vi "MTMount_getNextSample_OSS6.vi"(8 "error in (no error)":errorcluster, 11 "OSS6_Ctl":T1) -> (0 "error out":errorcluster, 2 "function return":i32, 3 "OSS6_Ctl out":T1)   [LabVIEW 2018, in "SALLV_MTMount.lvlib"]
doc: "int MTMount_shm_getNextSample_OSS6LV(MTMount_OSS6LV *OSS6_Ctl );"
uses:
  SALLV_MTMount.lvlib
  DataTypes/OSS6.ctl
  SALLV_MTMount.so
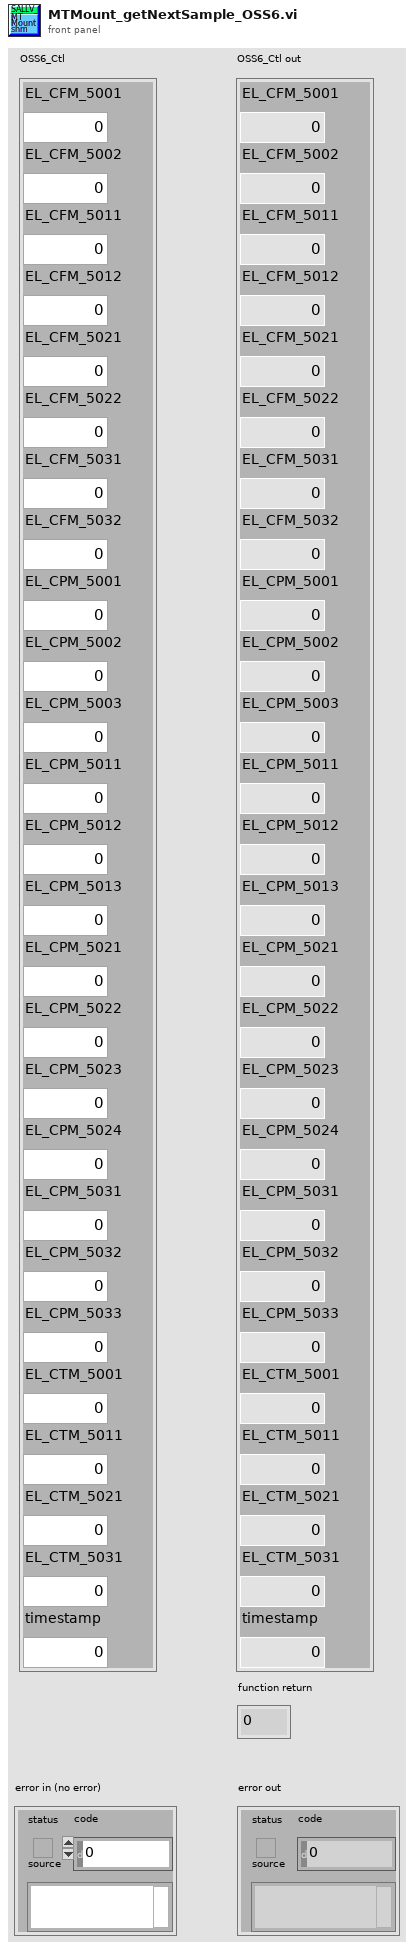
[diagram p1: front panel]
types:
  T1 = typedef "SALLV_MTMount.lvlib/OSS6.ctl" = cluster{"EL_CFM_5001":dbl, "EL_CFM_5002":dbl, "EL_CFM_5011":dbl, "EL_CFM_5012":dbl, "EL_CFM_5021":dbl, "EL_CFM_5022":dbl, "EL_CFM_5031":dbl, "EL_CFM_5032":dbl, "EL_CPM_5001":dbl, "EL_CPM_5002":dbl, "EL_CPM_5003":dbl, "EL_CPM_5011":dbl, "EL_CPM_5012":dbl, "EL_CPM_5013":dbl, "EL_CPM_5021":dbl, "EL_CPM_5022":dbl, "EL_CPM_5023":dbl, "EL_CPM_5024":dbl, "EL_CPM_5031":dbl, "EL_CPM_5032":dbl, "EL_CPM_5033":dbl, "EL_CTM_5001":dbl, "EL_CTM_5011":dbl, "EL_CTM_5021":dbl, "EL_CTM_5031":dbl, "timestamp":dbl}
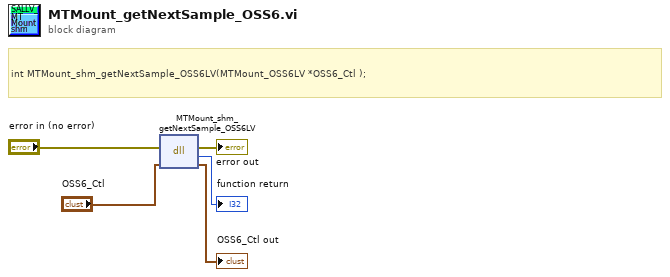
[diagram p0: block diagram]
diagram:
  # "int MTMount_shm_getNextSample_OSS6LV(MTMount_OSS6LV *OSS6_Ctl );"
  n1 = dll-call lib="home/ttsai/Document/salApiMTMount/SALLV_MTMount/SALLV_MTMount.*" fn="MTMount_shm_getNextSample_OSS6LV"(error in="error in (no error)", "OSS6_Ctl"="OSS6_Ctl") -> (error out=→"error out":errorcluster, →"function return":i32, "OSS6_Ctl"=→"OSS6_Ctl out":T1)  [unwired: 2 in, 1 out]
